vi "170729-uEye_Trigger_8bit-BM.vi"(6 "error in":errorcluster, 7 "Frame rate":dbl(slide)=20.0 min=1.0 max=100.0 step=1.0 scale=1.0..100.0 scale format="%^#_3g", 8 "Phase":u16=2, 9 "Save Path":path=path "C:/Users/SK-exp1/Desktop/tmp/BM") -> (0 "error out":errorcluster caption="error", 1 "DupFiles":bool)   [LabVIEW 2013]
doc: "SingleCapture_8bit nimmt ein Bilder von der Kamera auf und zeigt dieses an."
uses:
  <vilib>/vision/Image Controls.llb/IMAQ Image.ctl
  <vilib>/Analysis/_algsub.llb/Real Vector Norm.vi
  <vilib>/Analysis/Matrix/Numeric/Conversions/Array To Matrix - RA.vi
  Global_InitEndSync.vi
  <vilib>/Utility/file.llb/Write To Spreadsheet File (string).vi
  <vilib>/Analysis/Matrix/NI_Matrix.lvlib
  <vilib>/Analysis/NI_AALPro.lvlib
  <vilib>/vision/NI_Vision_Development_Module.lvlib
panel:
  in  "Threshold Limits":cluster{"Lower value":u8, "Upper value":u8}={"Lower value"=110, "Upper value"=255} {"Upper value" step=1 scale=0.0..255.0; "Lower value" step=1 scale=0.0..255.0}
  in  "Settings":T1={"Objects"=1, "Threshold"=250, "Reject Border"=FALSE, "Fill Holes"=FALSE, "Min Object Size"=TRUE, "Min Size"=150, "Max Object Size"=FALSE, "Max Size"=2000, "Show Search Area"=FALSE, "Show Center"=FALSE, "Show Bounding Box"=FALSE} {"Objects" items=["Bright Objects", "Dark Objects"]; "Threshold" min=1 max=999999999 step=1; "Max Size" min=1 max=999999999 step=1; "Min Size" min=1 max=999999999 step=1}
  out "REC & Tracking State":string
  out "appended path":path
  in  "ROI to track":T2={"Left"=207, "Top"=205, "Right"=287, "Bottom"=285, "Rotation"=0.0} {"Rotation" format="%.2f"; "Left" scale=0.0..1024.0; "Right" scale=0.0..1024.0}
  out "Tracking":T3(plugin-control)
  in  "Shape Adapted Mean Shift ?":bool
  in  "Mean Shift Options in":T4={"Number of Histogram Bins"=10, "Blending Parameter (%)"=20.0, "Max Scale Change (%)"=0.0, "Max Rotation Change  (0-180 degree)"=90.0, "Max Shape Change (%)"=20.0, "Maximum Iterations"=20}
  out "Video":u8[][](graph)
  in  "Online Parameter Setting?":bool
  in  "Exposure":bool
  in  "Gamma":i32(slide) min=0 max=1000 step=100 scale=0.0..1000.0
  in  "Gamma":bool
  in  "Blacklevel Offset":i32(slide)=255 min=0 max=255 scale=0.0..255.0
  in  "Exposure Time":dbl(slide)=66.62091228070176 min=0.008982456140350877 max=66.62091228070176 step=0.05487719298245614 scale=0.008982456140350877..66.62091228070176 scale format="%#.3g"
  in  "Edge Filter Enable / Disable":bool
  in  "Edge Filter":i32(ring)=2 items=["High"=1, "Low"=2]
  in  "Blacklevel Compensation":bool
  in  "Hotpixel correction":bool
  in  "Master Gain":i32(slide)=100 min=0 max=100 scale=0.0..100.0
  in  "Autogain":bool
  in  "Load Parameter?":bool=TRUE
  in  "Parameter Path":path=path "C:/Users/SK-exp1/Desktop/CamSetting/CamParam-190305-2-BM.ini"
  out "FPS":dbl=46.51595497255558
  in  "Camera ID":u32
  out "Get Trigger Mode":u16(ring)=4097 items=["Off"=0, "Hi-Low"=4097, "Low-Hi"=4098, "Software"=4104]
  in  "Trigger Mode":i32(ring)=4097 items=["IS_SET_TRIGGER_OFF"=0, "IS_SET_TRIGGER_HI_LO"=4097, "IS_SET_TRIGGER_LO_HI"=4098, "IS_SET_TRIGGER_SOFTWARE"=4104, "IS_GET_EXTERNALTRIGGER"=32768, "IS_GET_TRIGGER_STATUS"=32769]
  out "Height":i32=500
  out "Width":i32=500
  out "Bits/Pixel":i32=8
  in  "REC Stop":bool
  # "Setting"
  # "Image information"
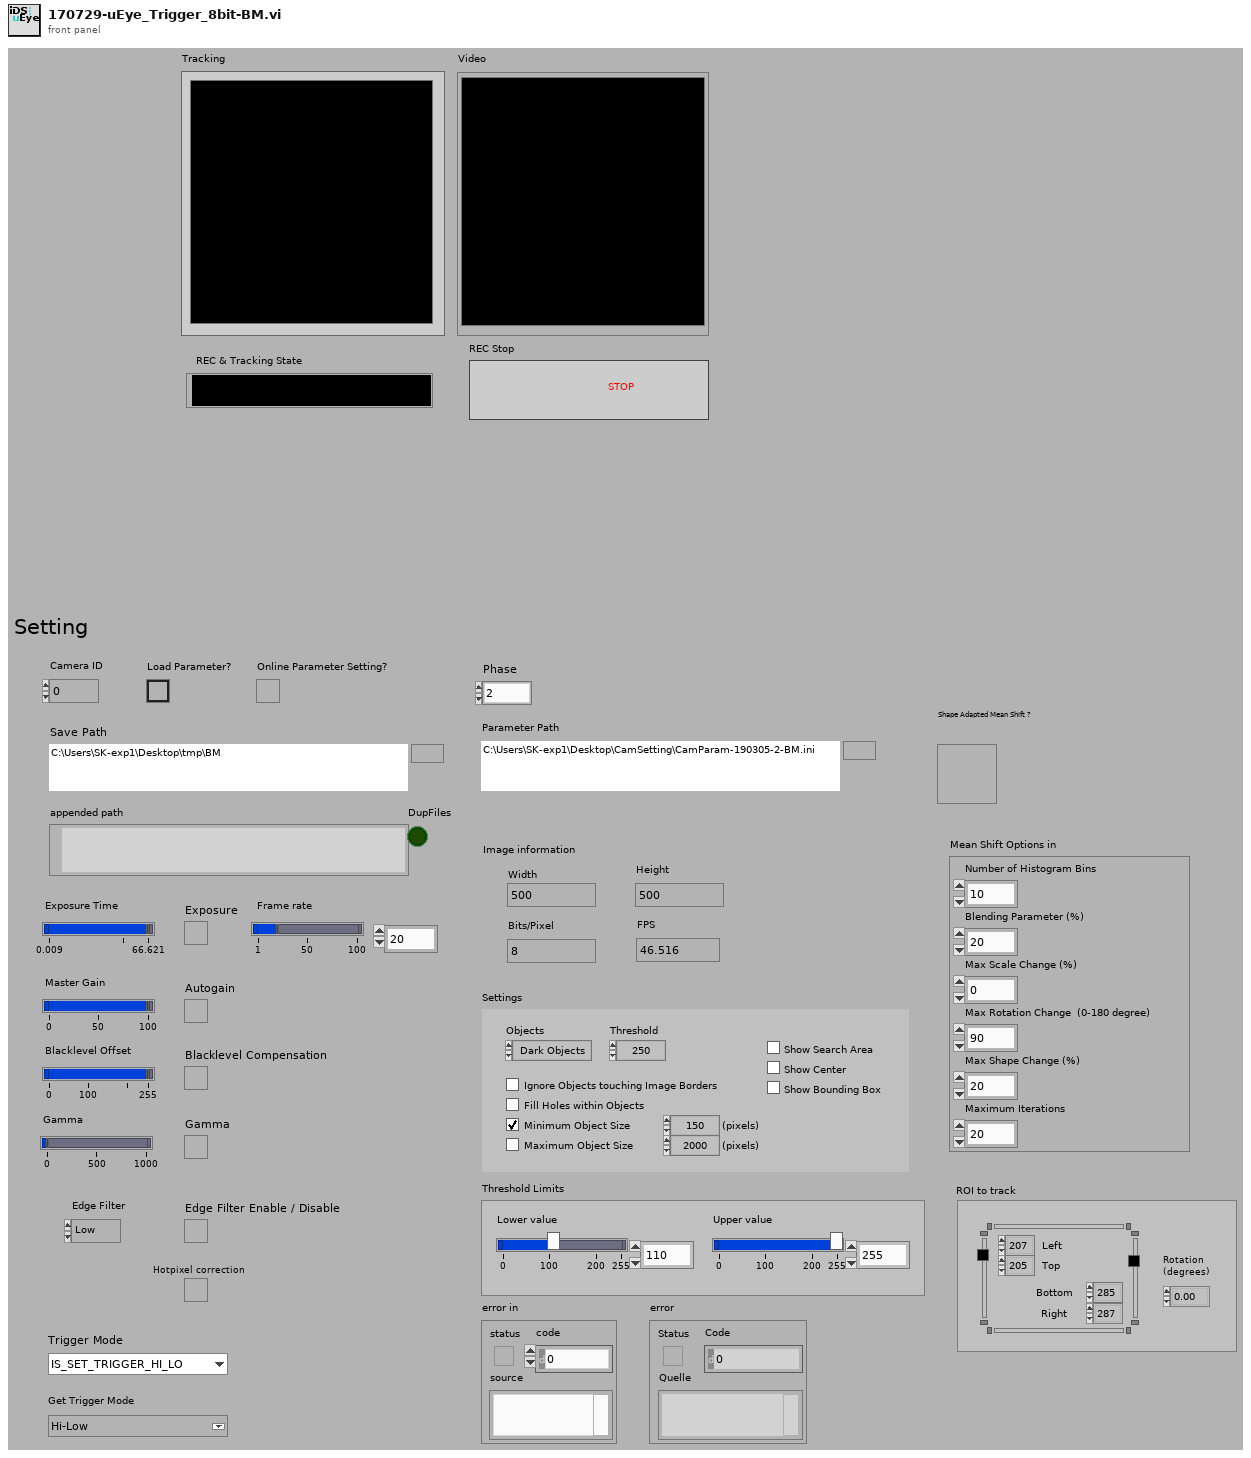
[diagram p1: front panel]
types:
  T1 = cluster{"Objects":u16, "Threshold":i32, "Reject Border":bool, "Fill Holes":bool, "Min Object Size":bool, "Min Size":i32, "Max Object Size":bool, "Max Size":i32, "Show Search Area":bool, "Show Center":bool, "Show Bounding Box":bool}
  T2 = typedef "IMAQ Rectangle" = cluster{"Left":i32, "Top":i32, "Right":i32, "Bottom":i32, "Rotation":dbl}
  T3 = typedef "IMAQ Image.ctl" = refnum<image>
  T4 = cluster{"Number of Histogram Bins":i32, "Blending Parameter (%)":dbl, "Max Scale Change (%)":dbl, "Max Rotation Change  (0-180 degree)":dbl, "Max Shape Change (%)":dbl, "Maximum Iterations":i32}
  T5 = typedef "IMAQ Object Tracking Session.ctl" = refnum<k20>
  T6 = cluster{"Number of Histogram Bins":i32, "Blending Parameter (%)":dbl, "Maximum Iterations":i32}
  T7 = typedef "IMAQ AVI2 Refnum.ctl" = refnum<k20>
  T8 = typedef "Image Type" = u32
  T9 = typedef "NI_Matrix.lvlib/RealMatrix.ctl" = dbl[][]
  T10 = typedef "ROI Descriptor" = cluster{"Global Rectangle":i32[], "Contours":cluster{"ID":enum32{"External", "Internal"}, "Type":u32, "Coordinates":i32[]}[]}
  T11 = cluster{"Label":string, "Score":i32, "Angle":dbl, "Location":cluster{"X":dbl, "Y":dbl}, "Bounding Box":cluster{"X":dbl, "Y":dbl}[], "Object Found?":bool}[]
  T12 = cluster{"Label":string, "Score":i32, "Angle":dbl, "Location":cluster{"X":dbl, "Y":dbl}, "Bounding Box":cluster{"X":dbl, "Y":dbl}[], "Object Found?":bool}
  T13 = cluster{"Object Center":cluster{"X":sgl, "Y":sgl}, "Bounding Box":cluster{"X Left":i32, "Y Top":i32, "X Right":i32, "Y Bottom":i32}, "Area":sgl, "Orientation":sgl, "Aspect Ratio":sgl, "Nb Holes":i32}[]
  T14 = cluster{"Object Center":cluster{"X":sgl, "Y":sgl}, "Bounding Box":cluster{"X Left":i32, "Y Top":i32, "X Right":i32, "Y Bottom":i32}, "Area":sgl, "Orientation":sgl, "Aspect Ratio":sgl, "Nb Holes":i32}
  T15 = cluster{"X Left":i32, "Y Top":i32, "X Right":i32, "Y Bottom":i32}
  T16 = cluster{"Left":i32, "Top":i32, "Right":i32, "Bottom":i32}
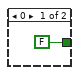
[diagram p2: hidden frame]
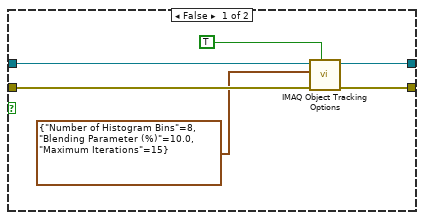
[diagram p3: hidden frame]
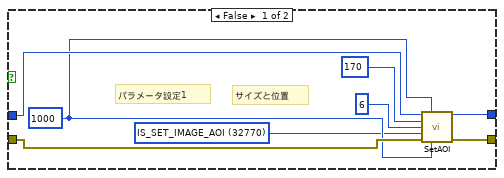
[diagram p5: hidden frame]
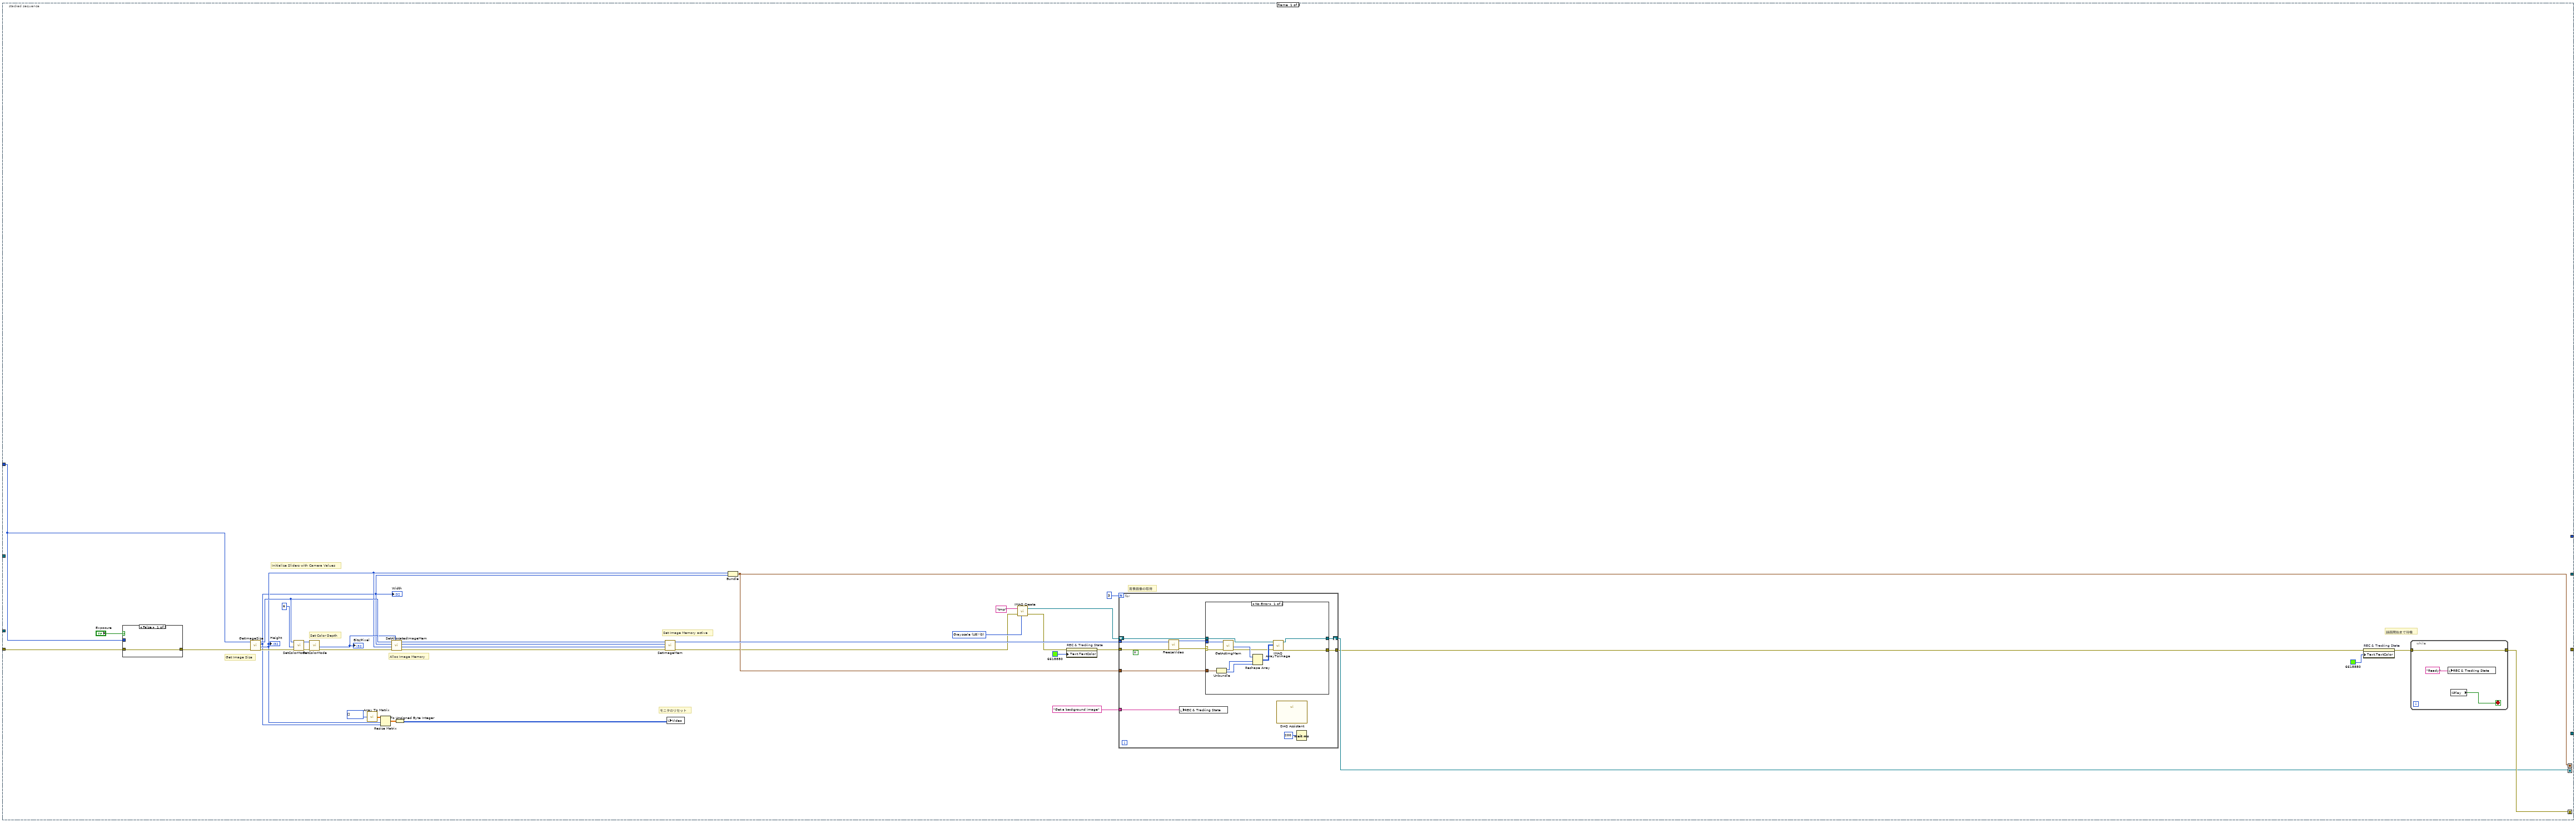
[diagram p7: hidden frame]
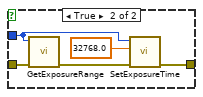
[diagram p9: hidden frame]
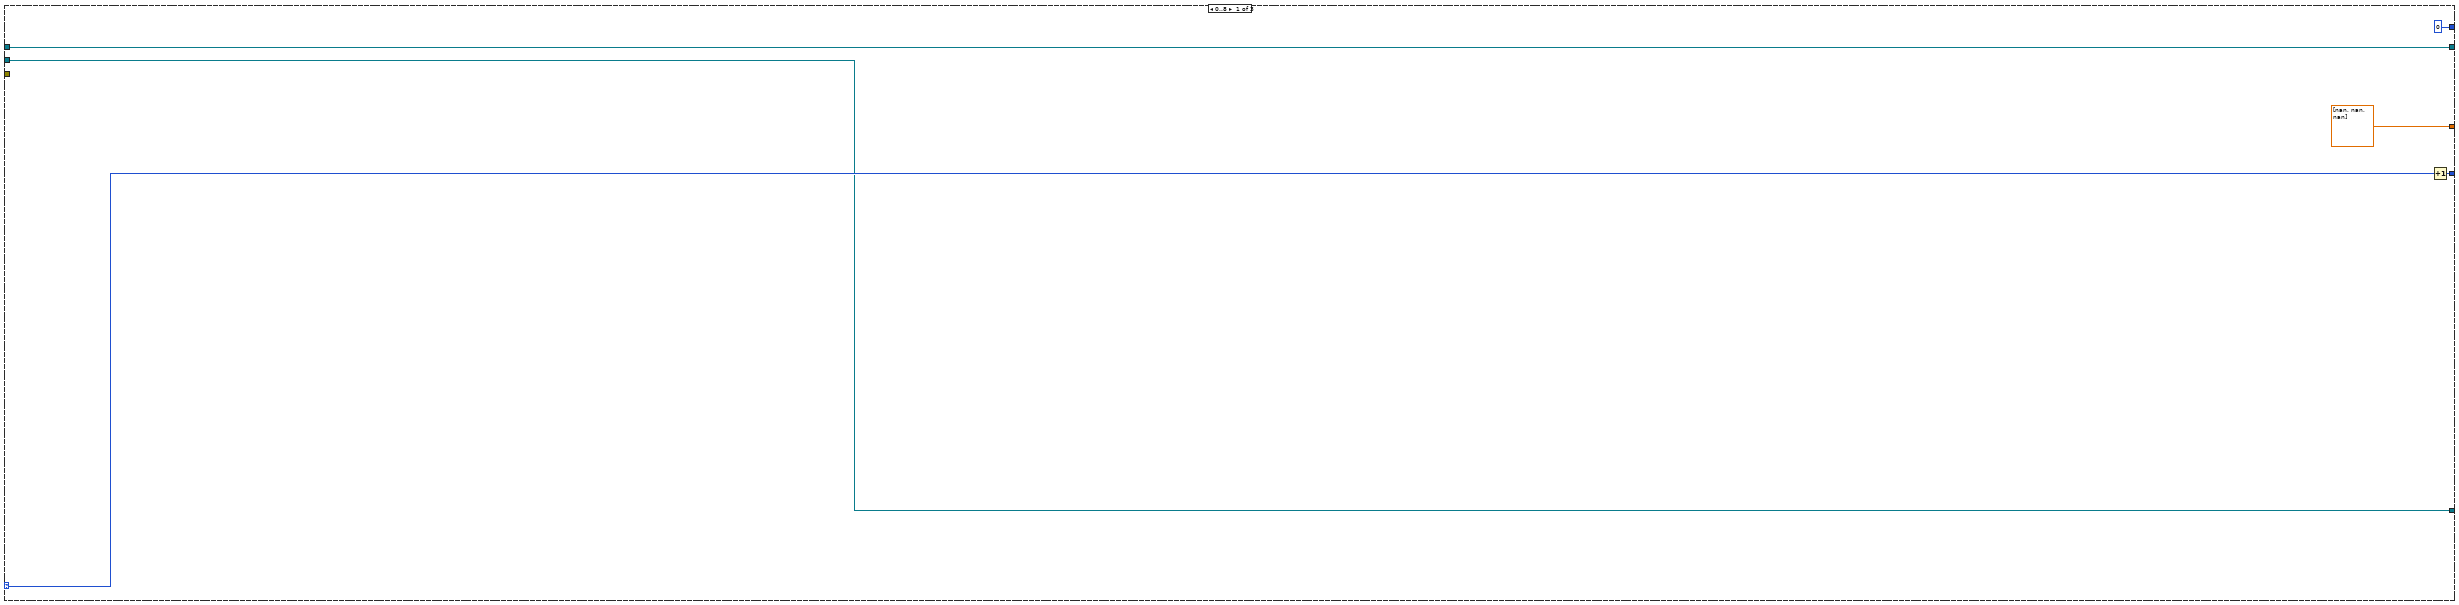
[diagram p11: hidden frame]
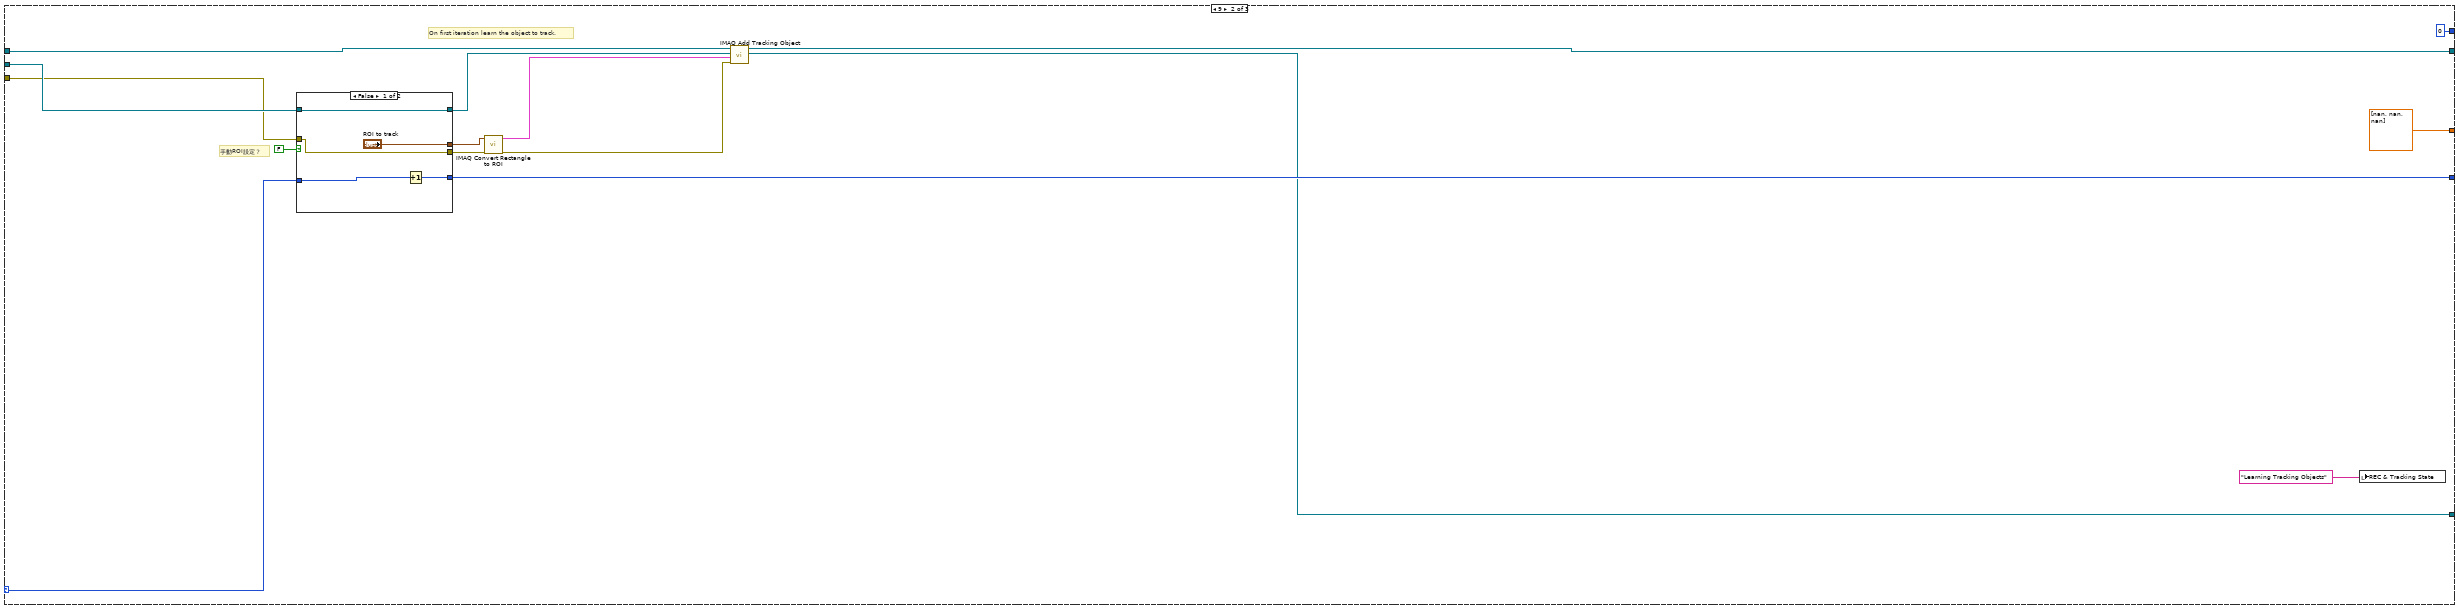
[diagram p12: hidden frame]
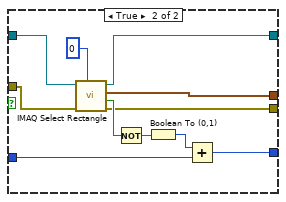
[diagram p13: hidden frame]
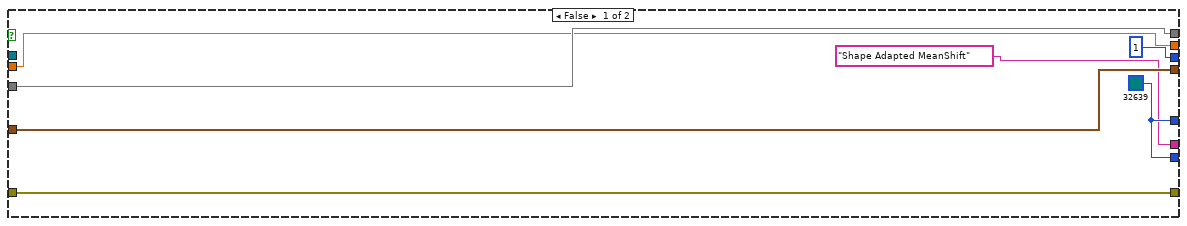
[diagram p14: hidden frame]
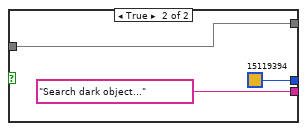
[diagram p15: hidden frame]
diagram:
  w9 = "xy"  # filename
  w8 = ".txt"  # format
  # "Initialize Camera"
  n1 = call <instrlib>:"InitCamera.vi"("Camera ID"="Camera ID") -> ("error out"=w26:errorcluster, "Camera Handle Out"=w27:u32)  [unwired: 9 in]
  n2 = case shown="True" "Load Parameter?" {
    tunnel: w27 -> [w36 w45]
    tunnel: [w29 w40] -> w1
    tunnel: w26 -> [w35 w44]
    tunnel: [w30 w39] -> w2
    frame False {
      w31 = 32770 items=["IS_SET_IMAGE_AOI"=32770, "IS_GET_IMAGE_AOI"=32771] ("Mode")
      w34 = 1000
      # "サイズと位置"
      # "パラメータ設定1"
      n3 = call <instrlib>:"SetAOI.vi"("Camera Handle In"=w36, "Width In"=w34, "XPos In"=170, "YPos In"=6, "Mode"=w31, "error in"=w35, "Height In"=w34) -> ("Camera Handle Out"=w29:u32, "error out"=w30:errorcluster)  [unwired: 3 in, 4 out]
    }
    frame True {
      w41 = 1 items=["IS_BINNING_DISABLE"=0, "IS_BINNING_2X_VERTICAL"=1, "IS_BINNING_2X_HORIZONTAL"=2, "IS_BINNING_4X_VERTICAL"=4, "IS_BINNING_4X_HORIZONTAL"=8, "IS_GET_BINNING"=32768, "IS_GET_SUPPORTED_BINNING"=32769] ("Mode")
      n4 = Path To String(path="Parameter Path") -> (string=w37:string)
      n5 = call <instrlib>:"LoadParameters.vi"("Camera Handle In"=w45, "Filename"=w37, "error in"=w44) -> ("Camera Handle Out"=w43:u32, "error out"=w42:errorcluster)  [unwired: 11 in]
      n6 = call <instrlib>:"SetBinning.vi"("error in"=w42, "Mode"=w41, "Camera Handle In"=w43) -> ("error out"=w39:errorcluster, "Camera Handle Out"=w40:u32)  [unwired: 6 in, 1 out]
    }
  }
  n7 = call "IMAQ Create Object Tracking Session"() -> ("error out"=w19:errorcluster, "Object Tracking Session"=w20:T5)  [unwired: 1 in, 9 out]
  n8 = case shown="True" "Shape Adapted Mean Shift ?" {
    tunnel: w20 -> [w48 w59]
    tunnel: w19 -> [w47 w58]
    tunnel: [w49 w57] -> w16
    tunnel: [w50 w56] -> w15
    frame False {
      n9 = call-poly "IMAQ Object Tracking Options"("Get/Set (Get)"=TRUE, "error in (no error)"=w47, "Mean Shift Options in"=T6 {"Number of Histogram Bins"=8, "Blending Parameter (%)"=10.0, "Maximum Iterations"=15}, "Object Tracking Session In"=w48) -> ("error out"=w49:errorcluster, "Object Tracking Session Out"=w50:T5)  [unwired: 5 in, 1 out]
    }
    frame True {
      n10 = local write "REC & Tracking State"("") -> ()
      n11 = call-poly "IMAQ Object Tracking Options"("Get/Set (Get)"=TRUE, "error in (no error)"=w58, "Shape Adapted Options in"="Mean Shift Options in", "Object Tracking Session In"=w59) -> ("error out"=w57:errorcluster, "Object Tracking Session Out"=w56:T5)  [unwired: 5 in, 1 out]
      n12 = local write "Tracking"(T3 refnum ("Tracking")) -> ()
    }
  }
  n13 = case shown="Default" "Phase" {
    tunnel: [_ w70] -> w14
    tunnel: "Save Path" -> [_ w67]
    tunnel: [_ w62] -> w10
    tunnel: [FALSE w61] -> w4
    frame 0 {
    }
    frame Default {
      w65 = "mv"  # filename
      w66 = ".avi"  # format
      n14 = call "AutoLinker.vi"("format"=w66, "filename"=w65, "Save Path"=w67) -> ("error out"=w63:errorcluster, "DupFiles"=w61:bool, "appended path"=w64:path)  [unwired: 6 in]
      "appended path" <- w64
      n15 = call "IMAQ AVI2 Create"("error in (no error)"=w63, "Codec"="Motion JPEG (NI Vision)", "Frames Per Second"="Frame rate", "AVI Path"=w64) -> ("error out"=w62:errorcluster, "AVI Refnum"=w70:T7)  [unwired: 6 in]
    }
  }
  n16 = call "AutoLinker.vi"("format"=w8, "filename"=w9, "Save Path"="Save Path") -> ("error out"=w6:errorcluster, "DupFiles"=w5:bool, "appended path"=w11:path)  [unwired: 6 in]
  n17 = Or(x=w4, y=w5) -> (x .or. y?=→"DupFiles":bool)
  n18 = Merge Errors(w2, w16, "error in", w10, w6) -> (w24:errorcluster)
  n19 = case shown="No Error" w24 {
    selector: w24 -> [w71 w79]
    tunnel: [w72 w82] -> w22
    tunnel: w1 -> [w72 w81]
    tunnel: [w71 w80] -> w23
    tunnel: [_ w78] -> w21
    tunnel: w14 -> [_ w77]
    tunnel: w15 -> [_ w76]
    tunnel: "Phase" -> [_ w75]
    tunnel: [_ w74] -> w13
    tunnel: w11 -> [_ w73]
    frame Error {
    }
    frame No Error {
      n20 = stacked-sequence {
        seq-local: [w97 _ _] -> [_ w161 _]
        seq-local: [w96 _ _] -> [_ w160 w480]
        seq-local: [w95 _ _] -> [_ w155 _]
        tunnel: w81 -> [w115 w159 w476]
        tunnel: [_ _ w472] -> w82
        tunnel: [_ _ w480] -> w80
        tunnel: w79 -> [w110 _ _]
        tunnel: [_ w158 _] -> w78
        tunnel: w77 -> [_ w157 _]
        tunnel: w76 -> [_ w154 _]
        tunnel: w75 -> [_ w156 _]
        tunnel: [_ w153 _] -> w74
        tunnel: w73 -> [_ w152 _]
        frame #0 {
          w91 = T8 0 items=["Grayscale (U8)", "Grayscale (I16)", "Grayscale (SGL)", "Complex (CSG)", "RGB (U32)", "HSL (U32)", "RGB (U64)", "Grayscale (U16)"] ("Image Type")
          # "背景画像の取得"
          # "モニタのリセット"
          # "録画開始まで待機"
          # "Initialize Sliders with Camera Values"
          # "Set Image Memory active"
          # "Alloc Image Memory"
          # "Set Color Depth"
          # "Get Image Size"
          n21 = case shown="False" "Exposure" {
            tunnel: w115 -> [_ w151]
            tunnel: w110 -> [w146 w149]
            tunnel: [w146 w147] -> w105
            frame False {
            }
            frame True {
              n22 = call <instrlib>:"GetExposureRange.vi"("error in"=w149, "Camera Handle In"=w151) -> ("error out"=w148:errorcluster)  [unwired: 5 in, 4 out]
              n23 = call <instrlib>:"SetExposureTime.vi"("error in"=w148, "Exposure Time"=32768.0, "Camera Handle In"=w151) -> ("error out"=w147:errorcluster)  [unwired: 6 in, 2 out]
            }
          }
          n24 = call <instrlib>:"GetImageSize.vi"("error in"=w105, "Camera Handle In"=w115) -> ("error out"=w109:errorcluster, "Height"=w102:i32, "Width"=w101:i32, "Camera Handle Out"=w116:u32)  [unwired: 6 in]
          "Width" <- w101
          "Height" <- w102
          n25 = call <instrlib>:"SetColorMode.vi"("error in"=w109, "Mode"=6, "Camera Handle In"=w116) -> ("error out"=w108:errorcluster, "Camera Handle Out"=w114:u32)  [unwired: 7 in]
          n26 = call <instrlib>:"GetColorMode.vi"("error in"=w108, "Camera Handle In"=w114) -> ("error out"=w107:errorcluster, "Bits/Pixel"=w112:i32)  [unwired: 6 in, 2 out]
          "Bits/Pixel" <- w112
          n27 = call-poly <vilib>:"Array To Matrix.vi"("Real 1D Array"=i32[] []) -> ("Real Matrix (Column Vector)"=w104:T9)
          n28 = Resize Matrix(1:w101, 2:w102, 4:w104) -> (0:w100:T9)
          n29 = call <instrlib>:"SetAllocatedImageMem.vi"("BitsPixel"=w112, "error in"=w107, "Height"=w102, "Width"=w101, "Camera Handle In"=w116) -> ("error out"=w111:errorcluster, "Image Memory Out"=w117:u8[], "Memory ID Out"=w118:i32, "Camera Handle Out"=w119:u32)  [unwired: 2 in, 1 out]
          n30 = To Unsigned Byte Integer(number=w100) -> (unsigned 8bit integer=w99:u8[][])
          n31 = call <instrlib>:"SetImageMem.vi"("error in"=w111, "Image Memory In"=w117, "Memory ID In"=w118, "Camera Handle In"=w119) -> ("error out"=w90:errorcluster, "Camera Handle Out"=w98:u32)  [unwired: 4 in, 2 out]
          n32 = local write "Video"(w99) -> ()
          n33 = Bundle("Height"=w102, "Width"=w101) -> (w97:cluster{"Height":i32, "Width":i32})  [unwired: 1 in]
          n34 = call "IMAQ Create"("Image Name"="tmp", "Image Type"=w91, "error in (no error)"=w90) -> ("New Image"=w93:T3, "error out"=w84:errorcluster)  [unwired: 2 in]
          n35 = property on="REC & Tracking State" class="Str"(error in=w84, "Text.TextColor"=u32 6618880 ("Color")) -> (error out=w83:errorcluster)  [unwired: 1 in, 1 out]
          n36 = for {
            N: 3 -> [_]
            tunnel: [w127] -> w88
            tunnel: w83 -> [w129]
            tunnel: w98 -> [w124]
            tunnel: w97 -> [w128]
            shift-right: [w126] -> w95
            shift-left: w93 -> [w125]
            tunnel: "Get a background image" -> [w120]
            (unwired) TRUE
            n37 = call <instrlib>:"FreezeVideo.vi"("error in"=w129, "Camera Handle In"=w124) -> ("error out"=w123:errorcluster, "Camera Handle Out"=w122:u32)  [unwired: 8 in]
            n38 = local write "REC & Tracking State"(w120) -> ()
            n39 = case shown="No Error" w123 {
              selector: w123 -> [w139 w141]
              tunnel: [w131 w142] -> w126
              tunnel: w125 -> [w132 w142]
              tunnel: w128 -> [w140 _]
              tunnel: w122 -> [w138 _]
              tunnel: [w130 w141] -> w127
              frame No Error {
                n40 = Unbundle(w140) -> ("Height"=w136:i32, "Width"=w135:i32)
                n41 = call <instrlib>:"GetActImgMem.vi"("error in"=w139, "Camera Handle In"=w138) -> ("error out"=w133:errorcluster, "Image Memory Out"=w137:u8[])  [unwired: 6 in, 2 out]
                n42 = Reshape Array(w137, w136, w135) -> (w134:u8[][])
                n43 = call "IMAQ ArrayToImage"("error in (no error)"=w133, "Image Pixels (U8)"=w134, "Image"=w132) -> ("error out"=w130:errorcluster, "Image Out"=w131:T3)  [unwired: 7 in]
              }
              frame Error {
              }
            }
            n44 = call "DAQ Assistant"() -> ()  [unwired: 18 in, 2 out]
            n45 = Wait (ms)(milliseconds to wait=200) -> ()  [unwired: 1 out]
          }
          n46 = property on="REC & Tracking State" class="Str"(error in=w88, "Text.TextColor"=u32 6618880 ("Color")) -> (error out=w87:errorcluster)  [unwired: 1 in, 1 out]
          n47 = while {
            tunnel: w87 -> [w144]
            tunnel: [w144] -> w96
            stop <- w145 stop-if-true
            n48 = local write "REC & Tracking State"("Ready") -> ()
            n49 = global read "Global_InitEndSync.vi" "Play"() -> (w145:bool)
          }
        }
        frame #1 {
          # "If Memory Allocation was successful start capture Video"
          n50 = case shown="No Error" w160 {
            tunnel: w159 -> [w192 _]
            tunnel: w161 -> [w193 _]
            tunnel: [w188 _] -> w158
            tunnel: w157 -> [w191 _]
            tunnel: w154 -> [w183 _]
            tunnel: w156 -> [w184 _]
            tunnel: w155 -> [w170 _]
            tunnel: [w181 _] -> w153
            tunnel: w152 -> [w177 _]
            frame No Error {
              w172 = T8 0 items=["Grayscale (U8)", "Grayscale (I16)", "Grayscale (SGL)", "Complex (CSG)", "RGB (U32)", "HSL (U32)", "RGB (U64)", "Grayscale (U16)"] ("Image Type")
              w174 = T8 4 items=["Grayscale (U8)", "Grayscale (I16)", "Grayscale (SGL)", "Complex (CSG)", "RGB (U32)", "HSL (U32)", "RGB (U64)", "Grayscale (U16)"] ("Image Type")
              w180 = T8 0 items=["Grayscale (U8)", "Grayscale (I16)", "Grayscale (SGL)", "Complex (CSG)", "RGB (U32)", "HSL (U32)", "RGB (U64)", "Grayscale (U16)"] ("Image Type")
              w182 = T8 0 items=["Grayscale (U8)", "Grayscale (I16)", "Grayscale (SGL)", "Complex (CSG)", "RGB (U32)", "HSL (U32)", "RGB (U64)", "Grayscale (U16)"] ("Image Type")
              n51 = property on="ROI to track" class="Clust (strict)"() -> ("Value"=w163:T2)  [unwired: 2 in, 2 out]
              n52 = Unbundle(w163) -> ("Left"=w164:i32, "Top"=w165:i32, "Right"=w166:i32, "Bottom"=w167:i32)  [unwired: 1 out]
              n53 = Build Array(w164, w165, w166, w167) -> (w162:i32[])
              n54 = call "IMAQ Create"("Image Name"="fore", "Image Type"=w182) -> ("New Image"=w185:T3)  [unwired: 3 in, 1 out]
              n55 = call "IMAQ Create"("Image Name"="mask", "Image Type"=w180) -> ("New Image"=w178:T3)  [unwired: 3 in, 1 out]
              n56 = call "IMAQ Create"("Image Name"="ForeMask", "Image Type"=w172) -> ("New Image"=w168:T3)  [unwired: 3 in, 1 out]
              n57 = call "IMAQ Create"("Image Name"="disp", "Image Type"=w174) -> ("New Image"=w175:T3)  [unwired: 3 in, 1 out]
              n58 = call "IMAQ Create"("Image Name"="frames") -> ("New Image"=w189:T3)  [unwired: 4 in, 1 out]
              n59 = while {
                tunnel: w193 -> [w228]
                tunnel: w192 -> [w194]
                tunnel: [w230] -> w188
                tunnel: w191 -> [w227]
                tunnel: w189 -> [w226]
                shift-right: [w210] -> _
                shift-left: 0 -> [w207]
                tunnel: w185 -> [w209]
                tunnel: w184 -> [w206]
                shift-right: [w204] -> w181
                shift-left: w183 -> [w203]
                tunnel: w178 -> [w202]
                tunnel: w177 -> [w201]
                tunnel: w175 -> [w200]
                tunnel: "Settings" -> [w199]
                tunnel: w170 -> [w198]
                tunnel: "Threshold Limits" -> [w197]
                tunnel: w168 -> [w196]
                tunnel: w162 -> [w195]
                i -> [w215]
                stop <- w218 stop-if-true
                w208 = 32769 items=["IS_SET_TRIG_OFF"=0, "IS_SET_TRIG_HI_LO"=1, "IS_SET_TRIG_LO_HI"=2, "IS_SET_TRIG_SOFTWARE"=8, "IS_SET_TRIGGER_HI_LO"=4097, "IS_SET_TRIGGER_LO_HI"=4098, "IS_SET_TRIGGER_SOFTWARE"=4104, "IS_GET_EXTERNALTRIGGER"=32768, "IS_GET_TRIGGER_STATUS"=32769] ("Trigger Mode")
                w225 = 32768 items=["IS_SET_TRIG_OFF"=0, "IS_SET_TRIG_HI_LO"=1, "IS_SET_TRIG_LO_HI"=2, "IS_SET_TRIG_SOFTWARE"=8, "IS_SET_TRIGGER_HI_LO"=4097, "IS_SET_TRIGGER_LO_HI"=4098, "IS_SET_TRIGGER_SOFTWARE"=4104, "IS_GET_EXTERNALTRIGGER"=32768, "IS_GET_TRIGGER_STATUS"=32769] ("Trigger Mode")
                # "ループタイミングの調節"
                n60 = call <instrlib>:"SetExternalTrigger.vi"("Trigger Mode"=w225, "Camera Handle In"=w194) -> ("error out"=w211:errorcluster, "Status"=w205:i32, "Camera Handle Out"=w212:u32)  [unwired: 7 in]
                "Get Trigger Mode" <- w205
                n61 = call <instrlib>:"SetExternalTrigger.vi"("error in"=w211, "Trigger Mode"=w208, "Camera Handle In"=w212) -> ("error out"=w213:errorcluster, "Camera Handle Out"=w214:u32)  [unwired: 6 in, 1 out]
                n62 = case shown="True" FALSE {
                  frame False {
                  }
                  frame True {
                    n63 = Wait Until Next ms Multiple(millisecond multiple=u32 10) -> ()  [unwired: 1 out]
                  }
                }
                n64 = Not Equal?(x="Trigger Mode", y=w205) -> (x != y?=w221:bool)
                n65 = call <instrlib>:"FreezeVideo.vi"("error in"=w213, "Camera Handle In"=w214) -> ("error out"=w216:errorcluster, "Camera Handle Out"=w217:u32)  [unwired: 8 in]
                n66 = Quotient & Remainder(x=w215, y=300) -> (x-y*floor(x/y)=w236:i32)  [unwired: 1 out]
                n67 = Equal To 0?(x=w236) -> (x = 0?=w235:bool)
                n68 = case shown="No Error" w216 {
                  selector: w216 -> [w284 _]
                  tunnel: [w292 w426] -> w230
                  tunnel: w228 -> [w291 _]
                  tunnel: w227 -> [w290 w426]
                  tunnel: w226 -> [w289 _]
                  tunnel: w217 -> [w288 _]
                  tunnel: w203 -> [w283 w424]
                  tunnel: [w279 w425] -> w210
                  tunnel: w207 -> [w280 w425]
                  tunnel: w209 -> [w263 _]
                  tunnel: w206 -> [w282 _]
                  tunnel: [w281 w424] -> w204
                  tunnel: w202 -> [w260 _]
                  tunnel: w201 -> [w276 _]
                  tunnel: w200 -> [w270 _]
                  tunnel: w199 -> [w259 _]
                  tunnel: w198 -> [w238 _]
                  tunnel: w197 -> [w240 _]
                  tunnel: w196 -> [w246 _]
                  tunnel: w195 -> [w245 _]
                  frame No Error {
                    # "追尾の成否"
                    # "Show Tracking Image"
                    # "リフト昇降状態"
                    # "Show Image"
                    n69 = call <instrlib>:"GetActImgMem.vi"("error in"=w284, "Camera Handle In"=w288) -> ("error out"=w261:errorcluster, "Image Memory Out"=w285:u8[])  [unwired: 6 in, 2 out]
                    n70 = Unbundle(w291) -> ("Height"=w287:i32, "Width"=w286:i32)
                    n71 = Reshape Array(w285, w287, w286) -> (w262:u8[][])
                    "Video" <- w262
                    n72 = call "IMAQ ArrayToImage"("error in (no error)"=w261, "Image Pixels (U8)"=w262, "Image"=w263) -> ("Image Out"=w237:T3)  [unwired: 7 in, 1 out]
                    n73 = call "IMAQ ArrayToImage"("error in (no error)"=w261, "Image Pixels (U8)"=w262, "Image"=w260) -> ("error out"=w256:errorcluster, "Image Out"=w255:T3)  [unwired: 7 in]
                    n74 = call "IMAQ Extract 2"("Optional Rectangle"=w245, "error in (no error)"=w256, "Image Src"=w255) -> ("error out"=w252:errorcluster, "Image Dst Out"=w254:T3)  [unwired: 7 in]
                    n75 = Array Subset(array=w245, length=2) -> (w249:i32[])  [unwired: 1 in]
                    n76 = call "IMAQ Subtract"("Image Src A"=w238, "Image Dst"=w246, "Image Src B"=w237, "error in (no error)"=w252) -> ("Image Dst Out"=w258:T3, "error out"=w257:errorcluster)  [unwired: 3 in]
                    n77 = call "IMAQ Inverse"("error in (no error)"=w257, "Image Src"=w258) -> ("error out"=w251:errorcluster, "Image Dst Out"=w253:T3)  [unwired: 8 in]
                    n78 = call "IMAQ ImageToImage 2"("Offset Left/Top"=w249, "error in (no error)"=w251, "Image Src (Small)"=w254, "Image Src (Large)"=w253) -> ("error out"=w241:errorcluster, "Image Dst Out"=w239:T3)  [unwired: 6 in]
                    n79 = call "IMAQ Threshold"("Replace Value"=sgl 255.0 ("Replace Value (1)"), "error in (no error)"=w241, "Range"=w240, "Image Src"=w239) -> ("error out"=w243:errorcluster, "Image Dst Out"=w244:T3)  [unwired: 6 in]
                    n80 = call "IMAQ NthOrder"("Image Src"=w244, "error in (no error)"=w243) -> ("Image Dst Out"=w248:T3, "error out"=w247:errorcluster)  [unwired: 5 in]
                    n81 = case shown="Default" w280 {
                      selector: w280 -> [w305 w318 w380]
                      tunnel: [w306 w321 w384] -> w281
                      tunnel: w283 -> [w306 w322 w383]
                      tunnel: w247 -> [_ w310 w351]
                      tunnel: [w301 w312 w369] -> w264
                      tunnel: [w304 w316 w365] -> w279
                      tunnel: [dbl[] [nan, nan, nan] ("Location") dbl[] [nan, nan, nan] ("Location") w366] -> w266
                      tunnel: w270 -> [_ _ w368]
                      tunnel: [0 0 w353] -> w268
                      tunnel: w248 -> [w301 w311 w342]
                      tunnel: w259 -> [_ _ w352]
                      frame 0..8 {
                        n82 = Increment(x=w305) -> (x+1=w304:i32)
                      }
                      frame 9 {
                        # "手動ROI設定？"
                        # "On first iteration learn the object to track."
                        n83 = case shown="False" FALSE {
                          tunnel: w311 -> [w326 w337]
                          tunnel: w318 -> [w327 w333]
                          tunnel: [w325 w332] -> w316
                          tunnel: [w326 w331] -> w307
                          tunnel: ["ROI to track" w330] -> w317
                          tunnel: w310 -> [w323 w329]
                          tunnel: [w323 w328] -> w309
                          frame False {
                            n84 = Increment(x=w327) -> (x+1=w325:i32)
                          }
                          frame True {
                            n85 = call "IMAQ Select Rectangle"("Window Number (0...15)"=0, "error in (no error)"=w329, "Image In"=w337) -> ("error out"=w328:errorcluster, "Cancelled"=w336:bool, "Rectangle"=w330:T2, "Image Out (duplicate)"=w331:T3)  [unwired: 5 in]
                            n86 = Not(x=w336) -> (.not. x?=w335:bool)
                            n87 = Boolean To (0,1)(Boolean=w335) -> (0, 1=w334:i16)
                            n88 = Add(x=w334, y=w333) -> (x+y=w332:i32)
                          }
                        }
                        n89 = call "IMAQ Convert Rectangle to ROI"("error in (no error)"=w309, "Rectangle"=w317) -> ("error out"=w308:errorcluster, "ROI Descriptor"=w320:T10)  [unwired: 7 in]
                        n90 = call "IMAQ Add Tracking Object"("error in (no error)"=w308, "ROI Descriptor"=w320, "Image"=w307, "Object Tracking Session In"=w322) -> ("Image (duplicate)"=w312:T3, "Object Tracking Session Out"=w321:T5)  [unwired: 1 in, 5 out]
                        n91 = local write "REC & Tracking State"("Learning Tracking Objects") -> ()
                      }
                      frame Default {
                        w339 = u32 2 items=["Frame", "Fill", "Highlight"] ("Drawing Mode (Frame)")
                        (unwired) u16 1 items=["Line", "Rectangle", "Oval"] ("Shape to draw")
                        # "追尾に成功したか OR \n中心からの距離が基準を超えていないか"
                        # "Get norm"
                        # "center"
                        # "radius + margin"
                        # "物体の位置座標と境界領域の抽出"
                        # "Track the object"
                        n92 = call "IMAQ Track Objects"("error in (no error)"=w351, "Image"=w342, "Object Tracking Session In"=w383) -> ("error out"=w363:errorcluster, "Objects (pixel)"=w372:T11, "Object Tracking Session Out"=w384:T5)  [unwired: 1 in, 5 out]
                        n93 = Index Array(array=w372) -> (element=w382:T12)  [unwired: 1 in]
                        n94 = Unbundle By Name(w382) -> ("Angle"=w361:dbl, "Location"=w381:cluster{"X":dbl, "Y":dbl}, "Bounding Box"=w360:cluster{"X":dbl, "Y":dbl}[])
                        n95 = Cluster To Array(cluster=w381) -> (array=w362:dbl[])
                        n96 = Subtract(x=w362, y=i32[] [245, 245]) -> (x-y=w377:dbl[])
                        n97 = call-poly <vilib>:"Vector Norm.vi"("norm type"=1, "Input Vector"=w377) -> ("norm"=w376:dbl)  [unwired: 8 in, 1 out]
                        n98 = Not A Number/Path/Refnum?(number/path/refnum=w376) -> (NaN/Path/Refnum?=w374:bool)
                        n99 = Greater?(x=w376, y=290) -> (0:w373:bool)
                        n100 = Or(x=w374, y=w373) -> (x .or. y?=w364:bool)
                        n101 = case shown="True" w364 {
                          tunnel: w363 -> [w391 w414]
                          tunnel: [w391 w413] -> w350
                          tunnel: w342 -> [_ w415]
                          tunnel: [w387 w392] -> w356
                          tunnel: [w389 w393] -> w358
                          tunnel: [w390 w397] -> w359
                          tunnel: w360 -> [w390 _]
                          tunnel: w362 -> [w389 _]
                          tunnel: [1 w417] -> w353
                          tunnel: ["Shape Adapted MeanShift" w416] -> w355
                          tunnel: [w387 w392] -> w354
                          tunnel: [w386 w408] -> w357
                          tunnel: w361 -> [w386 _]
                          tunnel: w352 -> [_ w406]
                          frame False {
                            w387 = u32 32639 ("Color")
                          }
                          frame True {
                            n102 = call "IMAQ Count Objects 2"("Settings"=w406, "error in (no error)"=w414, "Image"=w415) -> ("error out"=w413:errorcluster, "Objects"=w412:T13)  [unwired: 4 in, 3 out]
                            n103 = Index Array(array=w412) -> (element=w411:T14)  [unwired: 1 in]
                            n104 = Unbundle By Name(w411) -> ("Object Center"=w409:cluster{"X":sgl, "Y":sgl}, "Bounding Box"=w410:T15, "Orientation"=w408:sgl)  [unwired: 1 out]
                            n105 = Unbundle(w410) -> ("X Left"=w405:i32, "Y Top"=w402:i32, "X Right"=w404:i32, "Y Bottom"=w403:i32)
                            n106 = Cluster To Array(cluster=w409) -> (array=w394:sgl[])
                            n107 = Bundle("X Left"=w405, "Y Bottom"=w403) -> (w398:cluster{"X Left":i32, "Y Bottom":i32})  [unwired: 1 in]
                            n108 = Bundle("X Left"=w405, "Y Top"=w402) -> (w401:cluster{"X Left":i32, "Y Top":i32})  [unwired: 1 in]
                            n109 = Bundle("X Right"=w404, "Y Top"=w402) -> (w400:cluster{"X Right":i32, "Y Top":i32})  [unwired: 1 in]
                            n110 = Bundle("X Right"=w404, "Y Bottom"=w403) -> (w399:cluster{"X Right":i32, "Y Bottom":i32})  [unwired: 1 in]
                            n111 = Build Array(w401, w400, w399, w398, w401) -> (w397:cluster{"X Left":i32, "Y Top":i32}[])
                            n112 = Equal To 0?(x=w394) -> (x = 0?=w407:bool[])
                            n113 = And Array Elements(Boolean array=w407) -> (logical AND=w396:bool)
                            n114 = Not(x=w396) -> (.not. x?=w395:bool)
                            n115 = case shown="False" w395 {
                              tunnel: ["LOST" "Search dark object..."] -> w416
                              tunnel: [u32 14966322 ("Color") u32 15119394 ("Color")] -> w392
                              tunnel: w394 -> [_ w421]
                              tunnel: [dbl[] [nan, nan] w421] -> w393
                              frame False {
                              }
                              frame True {
                              }
                            }
                            n116 = Boolean To (0,1)(Boolean=w395) -> (0, 1=w417:i16)
                          }
                        }
                        "REC & Tracking State" <- w355
                        n117 = property on="ROI to track" class="Clust (strict)"(error in=w350) -> (error out=w343:errorcluster, "Value"=w349:T2)  [unwired: 1 in, 1 out]
                        n118 = Unbundle(w349) -> ("Left"=w348:i32, "Top"=w347:i32, "Right"=w346:i32, "Bottom"=w345:i32)  [unwired: 1 out]
                        n119 = Bundle("Left"=w348, "Top"=w347, "Right"=w346, "Bottom"=w345) -> (w344:T16)  [unwired: 1 in]
                        n120 = call "IMAQ Overlay Rectangle"("error in (no error)"=w343, "Drawing Mode (Frame)"=w339, "Rectangle"=w344, "Image"=w342) -> ("error out"=w340:errorcluster, "Image Out"=w341:T3)  [unwired: 6 in]
                        n121 = call "IMAQ Overlay Multiple Lines 2"("Image"=w341, "Line End Points"=w359, "Color"=w354, "error in (no error)"=w340, "Width"=5) -> ("Image Out"=w371:T3, "error out"=w370:errorcluster)  [unwired: 9 in]
                        n122 = Insert Into Array(array=w358, new element=w357) -> (w366:dbl[])  [unwired: 1 in]
                        n123 = property on="REC & Tracking State" class="Str"("Text.TextColor"=w356) -> ()  [unwired: 2 in, 2 out]
                        n124 = call "IMAQ Merge Overlay"("error in (no error)"=w370, "Image Dst"=w368, "Image Src"=w371) -> ("Image Dst Out"=w369:T3)  [unwired: 7 in, 1 out]
                        n125 = Increment(x=w380) -> (x+1=w365:i32)
                      }
                    }
                    "Tracking" <- w264
                    n126 = call "DAQ Assistant2"() -> ("data"=w273:bool[])  [unwired: 17 in, 2 out]
                    n127 = Index Array(array=w273) -> (element=w272:bool)  [unwired: 1 in]
                    n128 = Boolean To (0,1)(Boolean=w272) -> (0, 1=w269:i16)
                    n129 = Build Array(w269, w268) -> (w267:i32[])
                    n130 = To Double Precision Float(number=w267) -> (double precision float=w265:dbl[])
                    n131 = Insert Into Array(array=w265, new element=w266) -> (w271:dbl[])  [unwired: 1 in]
                    n132 = Number To Decimal String(number=w271) -> (decimal integer string=w274:string[])  [unwired: 1 in]
                    n133 = case shown="1, 2, Default" w282 {
                      tunnel: [w293 w300] -> w292
                      tunnel: w290 -> [w293 w299]
                      tunnel: w289 -> [_ w298]
                      tunnel: w261 -> [_ w297]
                      tunnel: w262 -> [_ w296]
                      frame 0 {
                      }
                      frame 1, 2, Default {
                        # "動画保存"
                        n134 = call "IMAQ ArrayToImage"("error in (no error)"=w297, "Image Pixels (U8)"=w296, "Image"=w298) -> ("error out"=w295:errorcluster, "Image Out"=w294:T3)  [unwired: 7 in]
                        n135 = call "IMAQ AVI2 Write Frame"("error in (no error)"=w295, "Image"=w294, "AVI Refnum"=w299) -> ("AVI Refnum (duplicate)"=w300:T7)  [unwired: 6 in, 2 out]
                      }
                    }
                    n136 = call-poly <vilib>:"Write To Spreadsheet File.vi"("transpose? (no:F)"=FALSE, "format (%s)"="%s", "append to file? (new file:F)"=TRUE, "1D data"=w274, "file path (dialog if empty)"=w276) -> ()  [unwired: 3 in, 1 out]
                  }
                  frame Error {
                  }
                }
                n137 = Quotient & Remainder(x=w215, y=300) -> (x-y*floor(x/y)=w233:i32)  [unwired: 1 out]
                n138 = Equal To 0?(x=w233) -> (x = 0?=w224:bool)
                n139 = And(x=w224, y="Online Parameter Setting?") -> (x .and. y?=w229:bool)
                n140 = case shown="True" w221 {
                  tunnel: w194 -> [_ w429]
                  tunnel: "Trigger Mode" -> [_ w428]
                  frame False {
                  }
                  frame True {
                    n141 = call <instrlib>:"SetExternalTrigger.vi"("Trigger Mode"=w428, "Camera Handle In"=w429) -> ()  [unwired: 7 in, 3 out]
                  }
                }
                n142 = case shown="True" w235 {
                  tunnel: w194 -> [_ w463]
                  frame False {
                  }
                  frame True {
                    n143 = call <instrlib>:"GetFramesPerSecond.vi"("Camera Handle In"=w463) -> ("FPS"=→"FPS":dbl)  [unwired: 8 in, 2 out]
                  }
                }
                n144 = case shown="True" w229 {
                  tunnel: w194 -> [_ w430]
                  frame False {
                  }
                  frame True {
                    # "パラメータ設定2"
                    # "Set Exposure Time"
                    n145 = call <instrlib>:"SetAutoParameter.vi"("enable"="Autogain", "Param"=34816, "Camera Handle In"=w430) -> ("Camera Handle Out"=w439:u32)  [unwired: 6 in, 2 out]
                    n146 = case shown="False" "Blacklevel Compensation" {
                      tunnel: w430 -> [w449 w452]
                      tunnel: "Blacklevel Offset" -> [w447 w450]
                      frame False {
                        n147 = call <instrlib>:"SetBlCompensation.vi"("Mode"=0, "offset"=w447, "Camera Handle In"=w449) -> ()  [unwired: 6 in, 3 out]
                      }
                      frame True {
                        n148 = call <instrlib>:"SetBlCompensation.vi"("Mode"=1, "offset"=w450, "Camera Handle In"=w452) -> ()  [unwired: 6 in, 3 out]
                      }
                    }
                    n149 = call <instrlib>:"SetExposureTime.vi"("Mode"=u16 32900, "Exposure Time"="Exposure Time", "Camera Handle In"=w430) -> ()  [unwired: 6 in, 3 out]
                    n150 = case shown="True" "Gamma" {
                      tunnel: w430 -> [_ w442]
                      frame False {
                      }
                      frame True {
                        n151 = call <instrlib>:"SetGamma.vi"("Gamma"="Gamma", "Camera Handle In"=w442) -> ()  [unwired: 8 in, 2 out]
                      }
                    }
                    n152 = case shown="True" "Edge Filter Enable / Disable" {
                      tunnel: w430 -> [w443 w446]
                      frame False {
                        n153 = call <instrlib>:"SetEdgeEnhancement.vi"("Mode"=0, "Camera Handle In"=w443) -> ()  [unwired: 8 in, 2 out]
                      }
                      frame True {
                        n154 = call <instrlib>:"SetEdgeEnhancement.vi"("Mode"="Edge Filter", "Camera Handle In"=w446) -> ()  [unwired: 8 in, 2 out]
                      }
                    }
                    n155 = case shown="True" "Hotpixel correction" {
                      tunnel: w430 -> [w454 w456]
                      frame False {
                        n156 = call <instrlib>:"SetHotPixelCorrection.vi"("Mode"=0, "Camera Handle In"=w454) -> ()  [unwired: 7 in, 3 out]
                      }
                      frame True {
                        n157 = call <instrlib>:"SetHotPixelCorrection.vi"("Mode"=2, "Camera Handle In"=w456) -> ()  [unwired: 7 in, 3 out]
                      }
                    }
                    n158 = case shown="True" "Autogain" {
                      tunnel: w439 -> [w457 w460]
                      frame False {
                        # "Set Master Gain"
                        n159 = call <instrlib>:"SetHardwareGain.vi"("Master Gain"="Master Gain", "Camera Handle In"=w457) -> ()  [unwired: 7 in, 3 out]
                      }
                      frame True {
                        # "On active AutoGain,\nset Master Gain Slider Value"
                        n160 = call <instrlib>:"SetHardwareGain.vi"("Mode"=32768, "Camera Handle In"=w460) -> ("Value"=w461:i32)  [unwired: 7 in, 2 out]
                        n161 = property on="Master Gain" class="Slide (strict)"("Value"=w461) -> ()  [unwired: 2 in, 2 out]
                      }
                    }
                  }
                }
                n162 = global read "Global_InitEndSync.vi" "Finish"() -> (w219:bool)
                n163 = Or(x=w219, y="REC Stop") -> (x .or. y?=w218:bool)
              }
            }
            frame Error {
              (unwired) ""
            }
          }
        }
        frame #2 {
          # "モニタのリセット"
          n164 = call <instrlib>:"GetImageSize.vi"("Camera Handle In"=w476) -> ("error out"=w468:errorcluster, "Height"=w474:i32, "Width"=w475:i32, "Camera Handle Out"=w469:u32)  [unwired: 7 in]
          n165 = call-poly <vilib>:"Array To Matrix.vi"("Real 1D Array"=i32[] []) -> ("Real Matrix (Column Vector)"=w479:T9)
          n166 = Resize Matrix(1:w475, 2:w474, 4:w479) -> (0:w477:T9)
          n167 = To Unsigned Byte Integer(number=w477) -> (unsigned 8bit integer=w473:u8[][])
          n168 = local write "Video"(w473) -> ()
          n169 = call <instrlib>:"GetActImgMem.vi"("error in"=w468, "Camera Handle In"=w469) -> ("error out"=w464:errorcluster, "Image Memory Out"=w465:u8[], "Memory Number"=w466:i32, "Camera Handle Out"=w467:u32)  [unwired: 6 in]
          n170 = call <instrlib>:"FreeImageMem.vi"("error in"=w464, "Image Memory"=w465, "Memory ID"=w466, "Camera Handle In"=w467) -> ("error out"=w470:errorcluster, "Camera Handle Out"=w471:u32)  [unwired: 6 in]
          n171 = call <instrlib>:"StopLiveVideo.vi"("error in"=w470, "Camera Handle In"=w471) -> ("Camera Handle Out"=w472:u32)  [unwired: 8 in, 1 out]
        }
      }
    }
  }
  n172 = flat-sequence {
    tunnel: w23 -> [w489]
    tunnel: w22 -> [w485]
    tunnel: w21 -> [w487]
    tunnel: "Phase" -> [w484]
    tunnel: w13 -> [w481]
    frame #0 {
      # "Free Image"
      # "Free Camera"
      n173 = call "IMAQ Dispose"("All Images? (No)"=TRUE, "error in (no error)"=w489) -> ("error out"=w486:errorcluster)  [unwired: 4 in]
      n174 = case shown="1, 2, Default" w484 {
        tunnel: w487 -> [_ w494]
        tunnel: w486 -> [w491 w493]
        tunnel: [w491 w492] -> w483
        frame 0 {
        }
        frame 1, 2, Default {
          # "Free AVI"
          n175 = call "IMAQ AVI2 Close"("error in (no error)"=w493, "AVI Refnum"=w494) -> ("error out"=w492:errorcluster)  [unwired: 9 in]
        }
      }
      n176 = call "IMAQ Dispose Object Tracking Session"("error in (no error)"=w483, "Object Tracking Session"=w481) -> ("error out"=w482:errorcluster)  [unwired: 9 in]
      n177 = call <instrlib>:"ExitCamera.vi"("error in"=w482, "Camera Handle In"=w485) -> ("error out"=→"error out":errorcluster)  [unwired: 9 in]
    }
    frame #1 {
      # "メモリ解放要求"
      n178 = local write "REC & Tracking State"("") -> ()
      n179 = Request Deallocation(TRUE ("メモリ開放要求？")) -> ()
      n180 = local write "Tracking"(T3 refnum ("Tracking")) -> ()
    }
  }
